vi "Set HDI Vacuum.vi"(8 "error in":errorcluster, 9 "On/Off":bool, 10 "Slot Number":i32, 11 "Gantry in":refnum<class "Gantry Class.lvclass">) -> (0 "error out":errorcluster, 3 "Gantry out":refnum<class "Gantry Class.lvclass">)   [LabVIEW 2011, in "Gantry Class.lvclass"]
uses:
  Gantry Class.lvclass
  WorkTable Class/WorkTable Class.lvclass
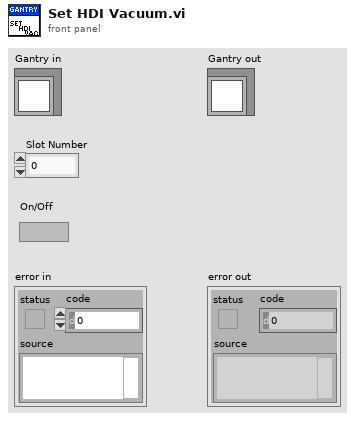
[diagram p1: front panel]
types:
  T1 = typedef "Worktable_HDI Slot.ctl" = cluster{"HDI Assembly State":enum16{"Empty", "Populated"}, "HDI Type":enum16{"HDI", "Polyimide"}, "Vacuum Channel":u32, "Location/Orientation":T2}
  T2 = typedef "Position_Orientation.ctl" = cluster{"Center":refnum<class "Vec3d Class.lvclass">, "Orientation":refnum<class "Orient3d Class.lvclass">}
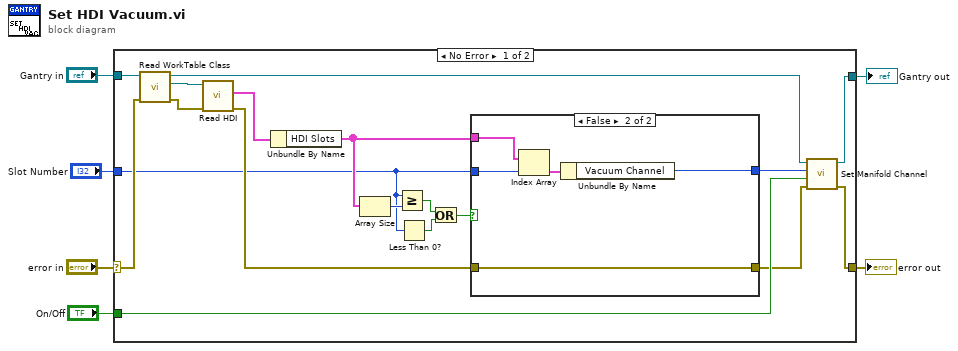
[diagram p0: block diagram]
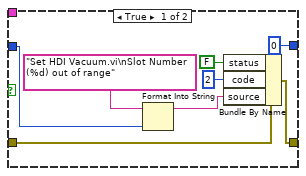
[diagram p2: hidden frame]
diagram:
  n1 = case shown="No Error" "error in" {
    selector: "error in" -> [w12 w39]
    tunnel: [w18 w39] -> w1
    tunnel: [w19 w38] -> w2
    tunnel: "Gantry in" -> [w24 w38]
    tunnel: "Slot Number" -> [w7 _]
    tunnel: "On/Off" -> [w22 _]
    frame No Error {
      n2 = call-dynamic "Read WorkTable Class.vi"("error in"=w12, "Gantry Class in"=w24) -> ("error out"=w13:errorcluster, "WorkTable Class.lvclass"=w17:refnum<class "WorkTable Class.lvclass">, "Gantry Class out"=w20:refnum<class "Gantry Class.lvclass">)  [unwired: 7 in]
      n3 = call-dynamic "Read HDI.vi"("error in (no error)"=w13, "WorkTable Class in"=w17) -> ("error out"=w11:errorcluster, "HDI"=w16:cluster{"HDI Slots":T1[]})  [unwired: 7 in, 1 out]
      n4 = Unbundle By Name(w16) -> ("HDI Slots"=w14:T1[])
      n5 = Array Size(array=w14) -> (size(s)=w15:i32)
      n6 = Greater Or Equal?(x=w7, y=w15) -> (x >= y?=w10:bool)
      n7 = Less Than 0?(x=w7) -> (x < 0?=w8:bool)
      n8 = Or(x=w10, y=w8) -> (x .or. y?=w9:bool)
      n9 = case shown="False" w9 {
        tunnel: w14 -> [_ w37]
        tunnel: w7 -> [w28 w36]
        tunnel: w11 -> [w27 w33]
        tunnel: [w26 w33] -> w21
        tunnel: [u8 0 ("Vacuum Channel") w34] -> w23
        frame True {
          n10 = Format Into String(format string="Set HDI Vacuum.vi\nSlot Number (%d) out of range" ("source"), w28) -> (resulting string=w29:string)  [unwired: 2 in, 1 out]
          n11 = Bundle By Name(cluster=w27, "status"=FALSE, "code"=2, "source"=w29) -> (w26:errorcluster)
        }
        frame False {
          n12 = Index Array(array=w37, index=w36) -> (element=w35:T1)
          n13 = Unbundle By Name(w35) -> ("Vacuum Channel"=w34:u32)
        }
      }
      n14 = call-dynamic "Set Manifold Channel.vi"("error in (no error)"=w21, "On/Off"=w22, "Manifold Channel"=w23, "Gantry Class in"=w20) -> ("error out"=w18:errorcluster, "Gantry Class out"=w19:refnum<class "Gantry Class.lvclass">)  [unwired: 6 in]
    }
    frame Error {
    }
  }
  "error out" <- w1
  "Gantry out" <- w2
